vi "01 MP_Reading a voltage.vi"() -> ()   [LabVIEW 2019]
uses:
  <vilib>/Instr/_visa.llb/VISA Configure Serial Port (Instr).vi
panel:
  out "Connected":bool
  in  "stop":bool
  in  "MicroPython code":string
  in  "MicroPython Port":refnum<visa-resource-name>
  out "Gauge":i32(knob) scale=0.0..1000.0
  # "Download and run the MicroPython code below\n\nSelect the Arduino port below\n\nHit the Run arrow and see the Gauge change to the value of the sensor (read over serial)"
  # "Hit Cmd E to see the diagram (code)"
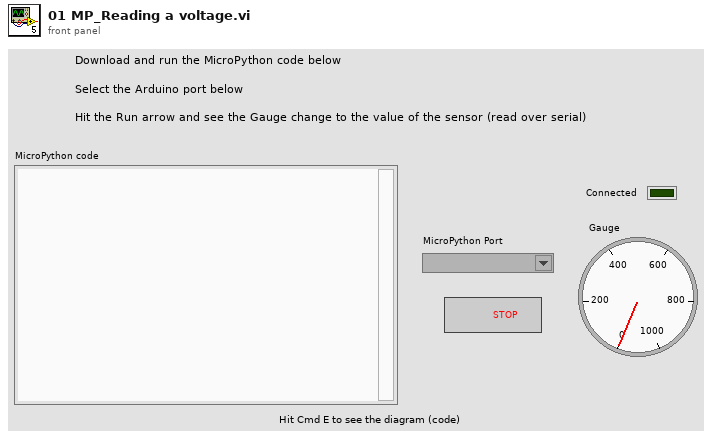
[diagram p1: front panel]
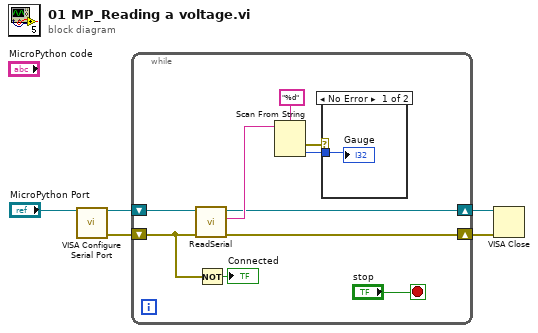
[diagram p0: block diagram]
diagram:
  n1 = call-poly "VISA Configure Serial Port"("VISA resource name"="MicroPython Port") -> ("VISA resource name out"=w4:refnum<visa-resource-name>, "error out"=w3:errorcluster)  [unwired: 13 in]
  n2 = while {
    shift-right: [w7] -> w1
    shift-left: w4 -> [w8]
    shift-right: [w6] -> w2
    shift-left: w3 -> [w9]
    stop <- "stop" stop-if-true
    n3 = call "ReadSerial.vi"("error in (no error)"=w9, "VISA Refnum in"=w8) -> ("error out"=w6:errorcluster, "String"=w10:string, "VISA Refnum out"=w7:refnum<visa-resource-name>)  [unwired: 7 in]
    n4 = Not(x=w9) -> (.not. x?=→"Connected":bool)
    n5 = Scan From String(format string="%d", input string=w10) -> (error out=w12:errorcluster, output 1=w11:i32)  [unwired: 3 in, 2 out]
    n6 = case shown="No Error" w12 {
      tunnel: w11 -> [w16 _]
      frame No Error {
        "Gauge" <- w16
      }
      frame Error {
      }
    }
  }
  n7 = VISA Close(VISA resource name=w1, error in (no error)=w2) -> ()  [unwired: 1 out]
